vi "Sort_Scen.vi"(1 "Scen in":T1(array[cluster])) -> (0 "Sorted Scen out":T1(array[cluster]))   [LabVIEW 2011]
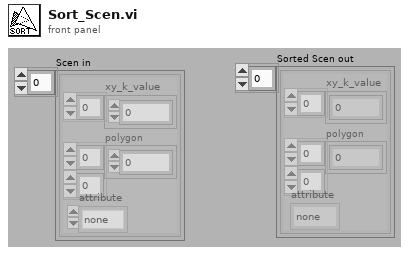
[diagram p1: front panel]
types:
  T1 = cluster{"xy_k_value":dbl[], "polygon":dbl[][], "attribute":enum16{"none", "transparent", "reflective", "white", "black", "grey", "red", "yellow", "green", "blue", "pink"}}[]
  T2 = cluster{"xy_angle":dbl[], "polygon":dbl[][], "attribute":u16}
  T3 = cluster{"xy_angle":dbl[], "polygon":dbl[][], "attribute":enum16{"none", "transparent", "reflective", "white", "black", "red", "yellow", "green", "blue", "pink"}}[]
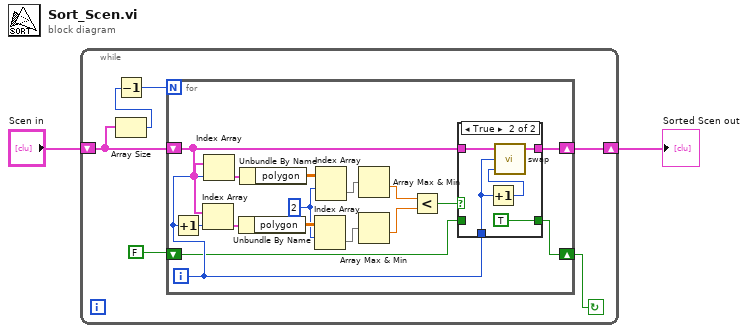
[diagram p0: block diagram]
diagram:
  n1 = while {
    shift-right: [w3] -> w1
    shift-left: "Scen in" -> [w6]
    stop <- w4 continue-if-true
    n2 = Array Size(array=w6) -> (size(s)=w7:i32)
    n3 = Decrement(x=w7) -> (x-1=w8:i32)
    n4 = for {
      N: w8 -> [_]
      shift-right: [w21] -> w4
      shift-left: FALSE -> [w19]
      shift-right: [w13] -> w3
      shift-left: w6 -> [w18]
      i -> [w20]
      w14 = 2 ("index")
      n5 = Increment(x=w20) -> (x+1=w24:i32)
      n6 = Index Array(array=w18, index=w24) -> (element=w23:T2)
      n7 = Index Array(array=w18, index=w20) -> (element=w22:T2)
      n8 = Unbundle By Name(w23) -> ("polygon"=w15:dbl[][])
      n9 = Unbundle By Name(w22) -> ("polygon"=w16:dbl[][])
      n10 = Index Array(array=w15, index (row)=w14) -> (element=w11:dbl[])  [unwired: 1 in]
      n11 = Index Array(array=w16, index (row)=w14) -> (element=w12:dbl[])  [unwired: 1 in]
      n12 = Array Max & Min(array=w12) -> (min value=w9:dbl)  [unwired: 3 out]
      n13 = Array Max & Min(array=w11) -> (min value=w10:dbl)  [unwired: 3 out]
      n14 = Less?(x=w9, y=w10) -> (x < y?=w17:bool)
      n15 = case shown="True" w17 {
        tunnel: [w26 TRUE] -> w21
        tunnel: w19 -> [w26 _]
        tunnel: w18 -> [w25 w29]
        tunnel: [w25 w30] -> w13
        tunnel: w20 -> [_ w28]
        frame False {
        }
        frame True {
          n16 = Increment(x=w28) -> (x+1=w27:i32)
          n17 = call "swap.vi"("index2"=w27, "index1"=w28, "Array_in"=w29) -> ("Array_out"=w30:T3)  [unwired: 2 in]
        }
      }
    }
  }
  "Sorted Scen out" <- w1
